vi "Servo MSMT Set Measurements.vi"(8 "error in (no error)":errorcluster, 11 "Servo MSMT in":refnum<class "Servo MSMT.lvclass">) -> (0 "error out":errorcluster, 3 "Servo MSMT out":refnum<class "Servo MSMT.lvclass">)   [LabVIEW 2018, in "Servo MSMT.lvlib" / "Servo MSMT.lvclass"]
uses:
  Servo MSMT.lvclass
  C:/Sequence Automation/Plugins/Measurement Interface.lvlibp/Measurement Interface.lvclass
  Servo MSMT.lvclass/Servo MSMT.ctl
  Read DC Pins.vi
  Read PAE Pins.vi
  Plugins/Measurement Interface.lvlibp/Private Methods/Measurement Parameters/Read Measurement Parameters.vi
  Plugins/String Database.lvlibp/String Database.lvclass
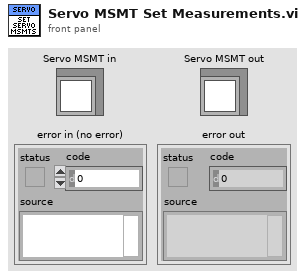
[diagram p1: front panel]
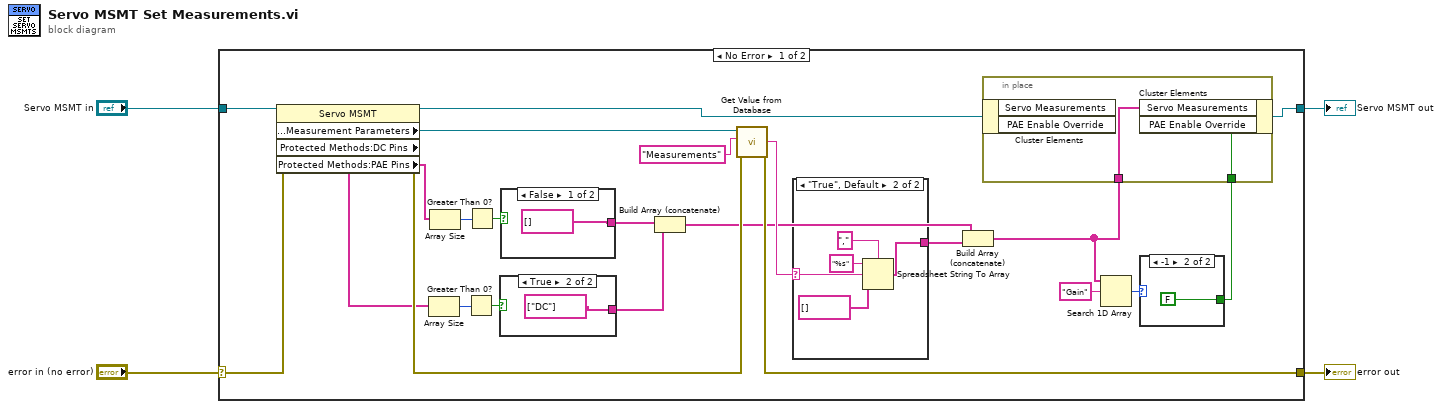
[diagram p0: block diagram]
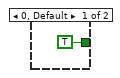
[diagram p2: hidden frame]
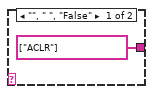
[diagram p3: hidden frame]
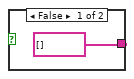
[diagram p4: hidden frame]
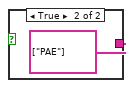
[diagram p5: hidden frame]
diagram:
  n1 = case shown="No Error" "error in (no error)" {
    selector: "error in (no error)" -> [w27 w43]
    tunnel: [w22 w43] -> w3
    tunnel: [w20 w42] -> w1
    tunnel: "Servo MSMT in" -> [w26 w42]
    frame No Error {
      n2 = property class="Servo MSMT"(reference=w26, error in=w27) -> (reference out=w21:refnum<class "Servo MSMT.lvclass">, error out=w23:errorcluster, "Protected Methods:Measurement Parameters"=w25:refnum<class "String Database.lvclass">, "Protected Methods:DC Pins"=w19:string[], "Protected Methods:PAE Pins"=w10:string[])
      n3 = Array Size(array=w19) -> (size(s)=w18:i32)
      n4 = Array Size(array=w10) -> (size(s)=w11:i32)
      n5 = Greater Than 0?(x=w18) -> (x > 0?=w17:bool)
      n6 = Greater Than 0?(x=w11) -> (x > 0?=w9:bool)
      n7 = case shown="True" w17 {
        tunnel: [string[] [] string[] ["DC"]] -> w12
        frame False {
        }
        frame True {
        }
      }
      n8 = case shown="False" w9 {
        tunnel: [string[] [] string[] ["PAE"]] -> w16
        frame False {
        }
        frame True {
        }
      }
      n9 = Build Array (concatenate)(w16, w12) -> (w14:string[])
      n10 = call "Get Value from Database.vi"("error in (no error)"=w23, "Entry Name"="Measurements", "Message in"=w25) -> ("error out"=w22:errorcluster, "Entry Value"=w15:string)  [unwired: 5 in, 2 out]
      n11 = case shown="\"True\", Default" w15 {
        selector: w15 -> [_ w34]
        tunnel: [string[] ["ACLR"] w32] -> w13
        frame "", " ", "False" {
        }
        frame "True", Default {
          n12 = Spreadsheet String To Array(delimiter (Tab)=",", format string="%s", spreadsheet string=w34, array type (2D Dbl)=string[] []) -> (array=w32:string[])
        }
      }
      n13 = Build Array (concatenate)(w14, w13) -> (w8:string[])
      n14 = Search 1D Array(1D array=w8, element="Gain") -> (index of element=w6:i32)  [unwired: 1 in]
      n15 = case shown="-1" w6 {
        tunnel: [TRUE FALSE] -> w5
        frame 0, Default {
        }
        frame -1 {
        }
      }
      n16 = in-place {
        in-place-border: w8 -> [w41]
        in-place-border: w5 -> [w40]
        n17 = in-place-cluster #1(w21) -> ()  [unwired: 2 out]
        n18 = in-place-cluster #1("Servo Measurements"=w41, "PAE Enable Override"=w40) -> (w20:refnum<class "Servo MSMT.lvclass">)
      }
    }
    frame Error {
    }
  }
  "error out" <- w3
  "Servo MSMT out" <- w1
